vi "file_counter_function.vi"(8 "error in (no error)":errorcluster, 11 "files_folder_path":path) -> (0 "error out":errorcluster, 2 "date searched":string, 3 "#files found":i32)   [LabVIEW 2015]
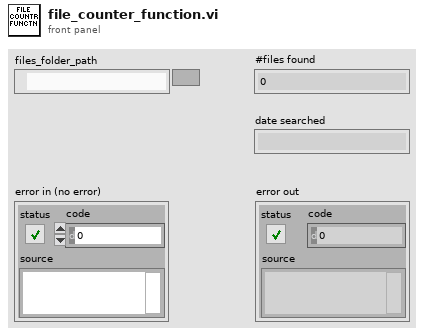
[diagram p1: front panel]
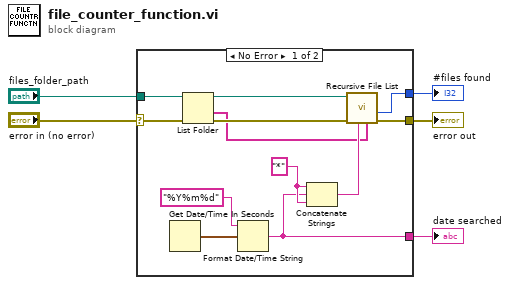
[diagram p0: block diagram]
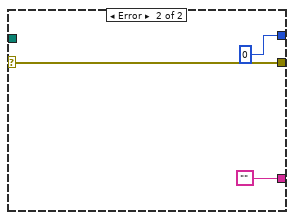
[diagram p2: hidden frame]
diagram:
  n1 = case shown="No Error" "error in (no error)" {
    selector: "error in (no error)" -> [w12 w19]
    tunnel: [w17 0 ("Number of Files")] -> w5
    tunnel: [w7 w19] -> w3
    tunnel: [w8 ""] -> w2
    tunnel: "files_folder_path" -> [w6 _]
    frame No Error {
      w13 = "*" ("string")
      n2 = Get Date/Time In Seconds() -> (seconds since 1Jan1904=w16:timestamp)
      n3 = List Folder(path=w6, error in=w12) -> (path out=w10:path, folder names=w9:string[], error out=w11:errorcluster)  [unwired: 2 in, 1 out]
      n4 = Format Date/Time String(time format string (%c)="%Y%m%d", seconds (now)=w16) -> (date/time string=w8:string)  [unwired: 1 in]
      n5 = Concatenate Strings(w13, w8, w13) -> (w14:string)
      n6 = call <vilib>:"Recursive File List.vi"("Folders to Exclude"=w9, "pattern"=w14, "error in (no error)"=w11, "Folder Path"=w10) -> ("error out"=w7:errorcluster, "Number of Files"=w17:i32)  [unwired: 3 in, 3 out]
    }
    frame Error {
    }
  }
  "#files found" <- w5
  "error out" <- w3
  "date searched" <- w2
